vi "Ping IP Address.vi"(8 "error in (no error)":errorcluster, 10 "IP Address":string="192.168.250.15") -> (0 "error out":errorcluster, 2 "Found?":bool)   [LabVIEW 2018]
panel:
  out "standard output":string
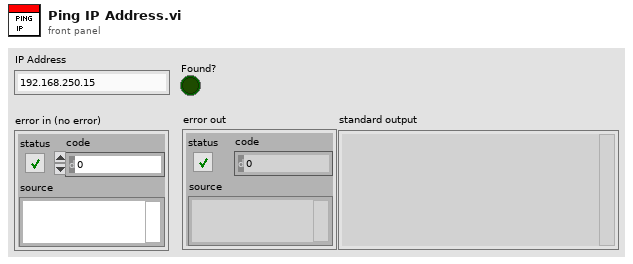
[diagram p1: front panel]
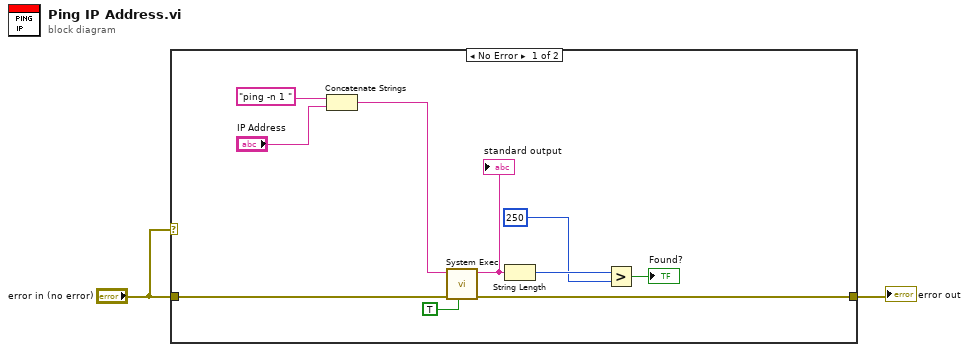
[diagram p0: block diagram]
diagram:
  n1 = case shown="No Error" "error in (no error)" {
    tunnel: "error in (no error)" -> [w10 w13]
    tunnel: [w6 w13] -> w1
    frame No Error {
      n2 = Concatenate Strings("ping -n 1 ", "IP Address") -> (w9:string)
      n3 = call <vilib>:"System Exec.vi"("run minimized? (F)"=TRUE, "error in (no error)"=w10, "command line"=w9) -> ("error out"=w6:errorcluster, "standard output"=w8:string)  [unwired: 5 in, 2 out]
      "standard output" <- w8
      n4 = String Length(string=w8) -> (length=w5:i32)
      n5 = Greater?(x=w5, y=250) -> (0:→"Found?":bool)
    }
    frame Error {
    }
  }
  "error out" <- w1
